vi "test2_V2.vi"() -> ()   [LabVIEW 2013]
uses:
  <vilib>/regexp/Match Regular Expression.xnode
panel:
  out "after match":string
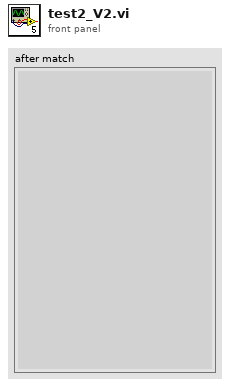
[diagram p1: front panel]
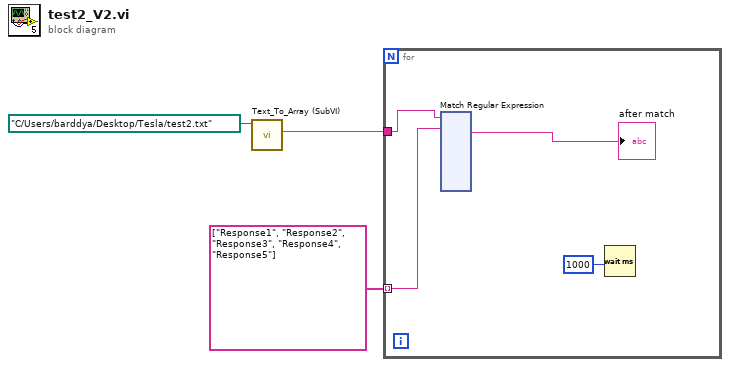
[diagram p0: block diagram]
diagram:
  n1 = call "Text_To_Array (SubVI).vi"("Path"=path "C:/Users/barddya/Desktop/Tesla/test2.txt" ("file path")) -> ("text"=w1:string)  [unwired: 8 in, 2 out]
  n2 = for {
    tunnel: string[] ["Response1", "Response2", "Response3", "Response4", "Response5"] -> [w5] mode=indexing
    tunnel: w1 -> [w7]
    n3 = xnode "Match Regular Expression"("input string"=w7, "regular expression"=w5) -> ("after match"=→"after match":string)  [unwired: 4 in, 9 out]
    n4 = Wait (ms)(milliseconds to wait=1000) -> ()  [unwired: 1 out]
  }
